vi "REPORT_AUDIT_prepare_results.vi"(11 "REPORT_AUDIT_all_info":T1) -> (3 "Array":string[][](array[string]))   [LabVIEW 2020]
uses:
  typedef/REPORT_AUDIT_all_info.ctl
  GEAR/typedef/REPORT_GEAR_statuses.ctl
  typedef/REPORT_AUDIT_control_index.ctl
  _misc/AULocalize/SubVIs/Get Localized Phrase Compact Interface 1D.vi
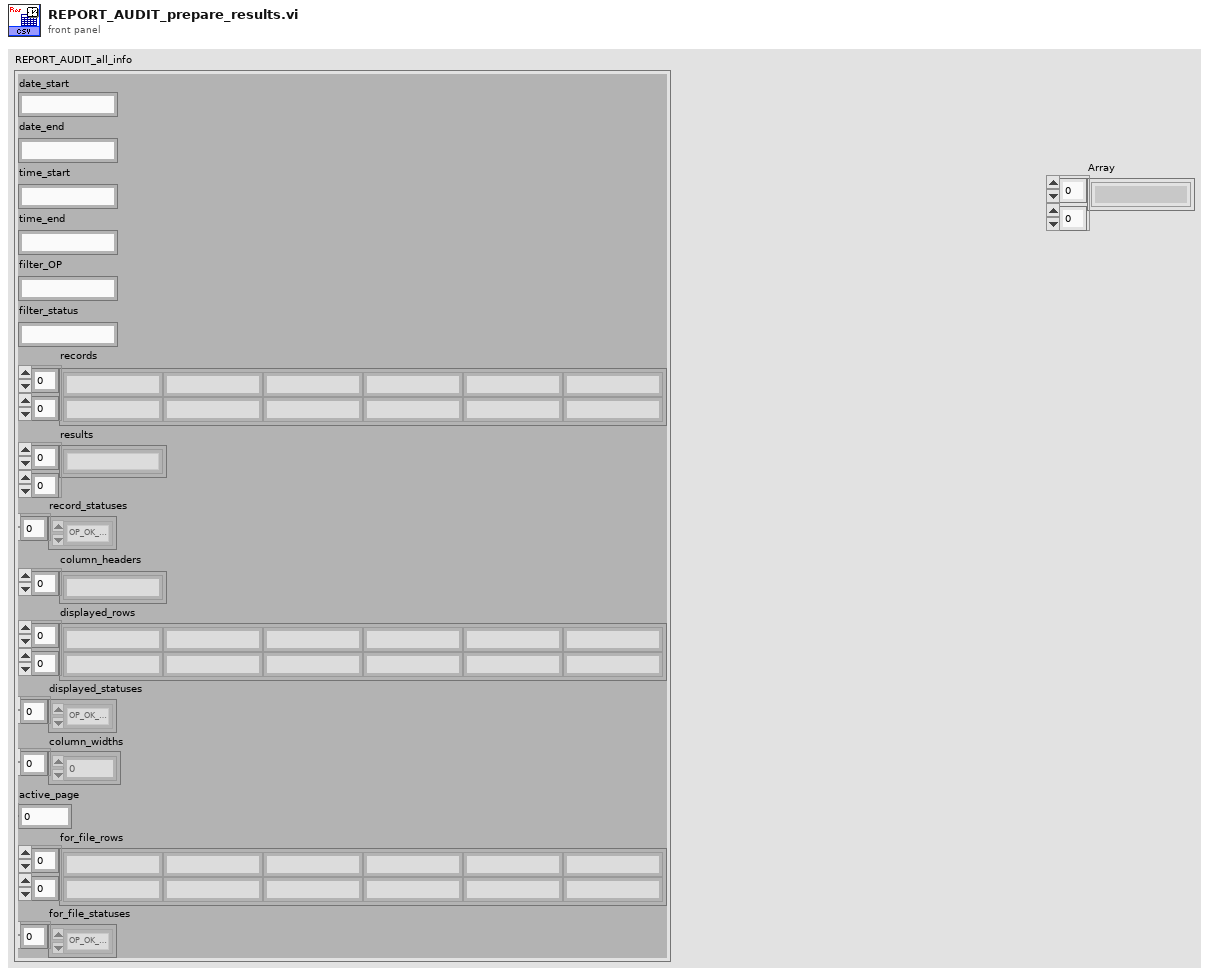
[diagram p1: front panel]
types:
  T1 = typedef "REPORT_AUDIT_all_info.ctl" = cluster{"date_start":string, "date_end":string, "time_start":string, "time_end":string, "filter_OP":string, "filter_status":string, "records":string[][], "results":string[][], "record_statuses":T2[], "column_headers":string[], "displayed_rows":string[][], "displayed_statuses":T2[], "column_widths":i16[], "active_page":i32, "for_file_rows":string[][], "for_file_statuses":T2[]}
  T2 = typedef "REPORT_GEAR_statuses.ctl" = enum16{"OP_OK_hide", "OP_OK_show", "OP_NOK_hide", "OP_NOK_show", "OP_interrupted_hide", "OP_interrupted_show", "OP_in_operation_hide", "OP_in_operation_show", "OP_unexpected_hide", "OP_unexpected_show", "RE_REAL_OK", "RE_REAL_NOK", "RE_STRING", "RE_sub_header", "RE_no_data", "RE_unexpected", "BA_sub_header", "BA_data", "BA_no_data"}
  T3 = typedef "REPORT_AUDIT_control_index.ctl" = enum16{"zeroing", "add_to_index", "get_index"}
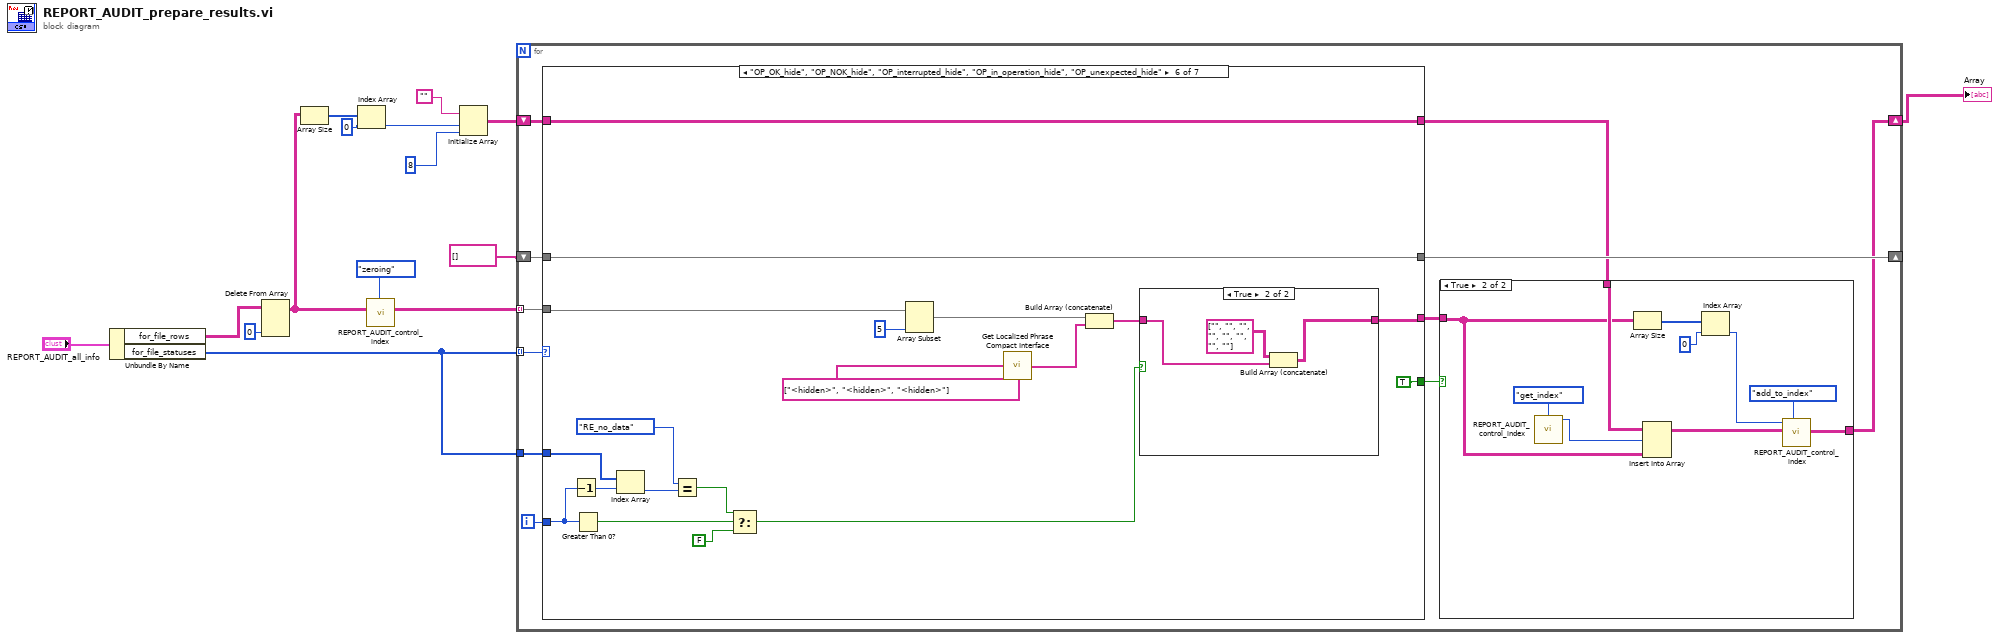
[diagram p0: block diagram]
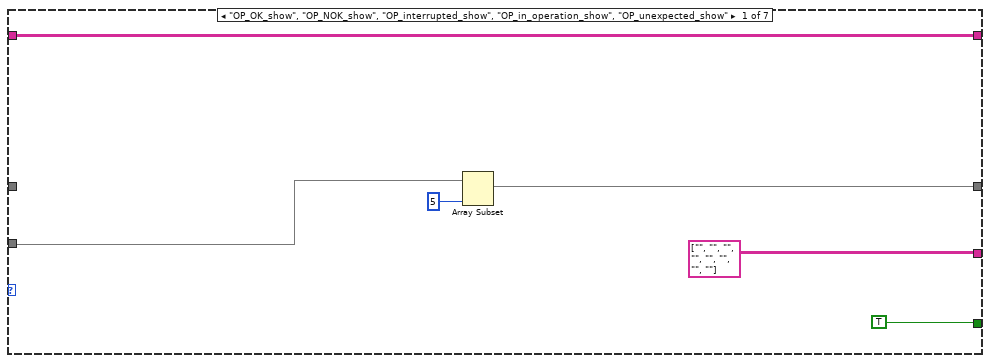
[diagram p3: hidden frame]
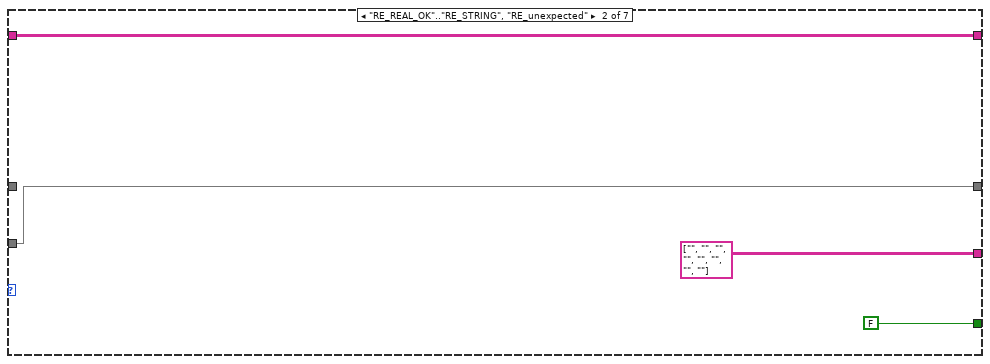
[diagram p4: hidden frame]
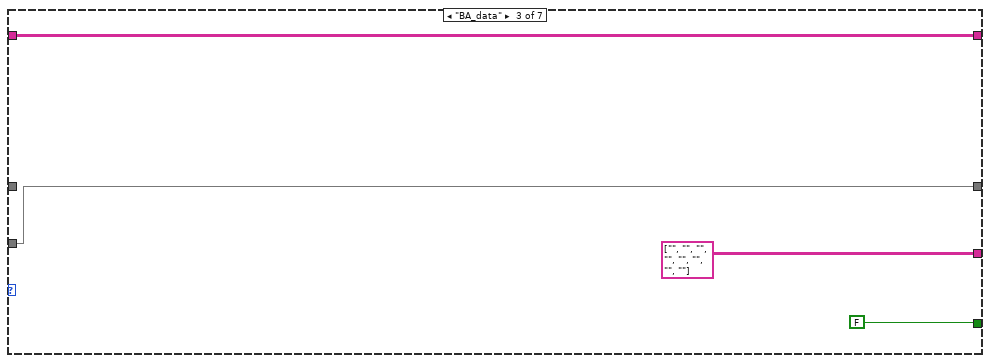
[diagram p5: hidden frame]
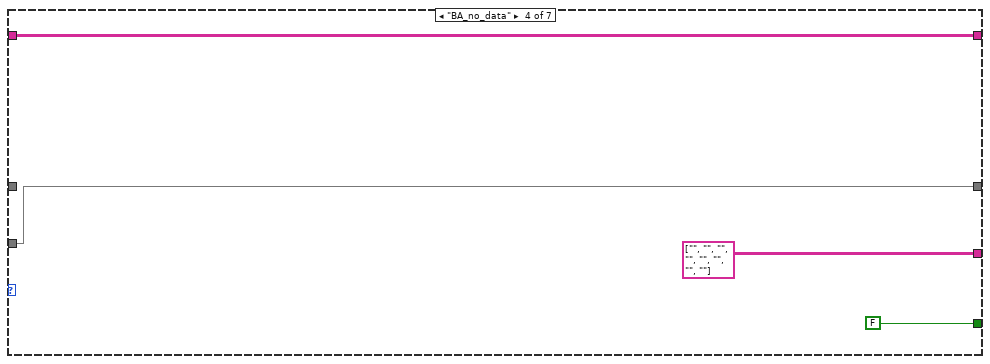
[diagram p6: hidden frame]
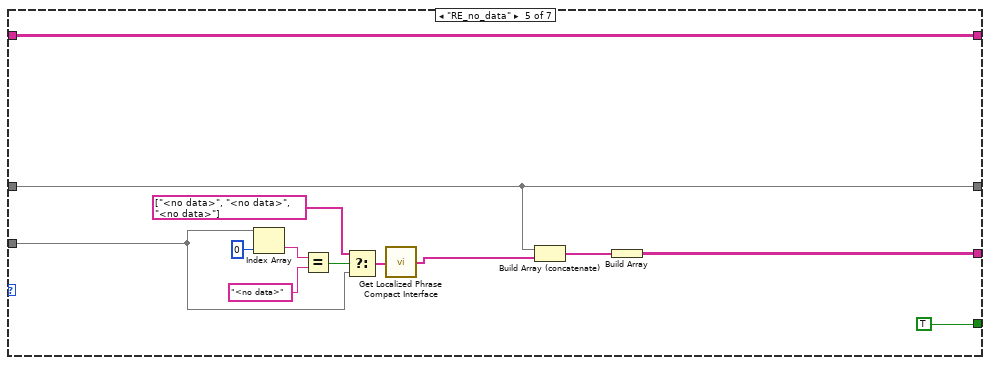
[diagram p7: hidden frame]
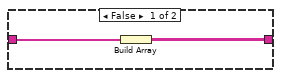
[diagram p8: hidden frame]
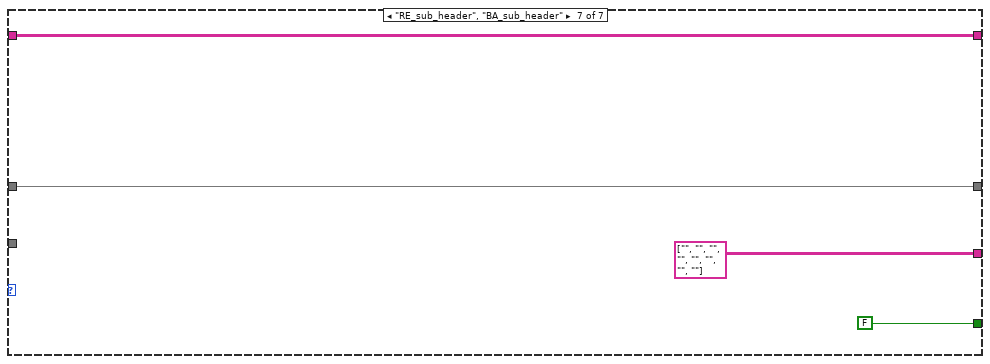
[diagram p9: hidden frame]
diagram:
  n1 = Unbundle By Name("REPORT_AUDIT_all_info") -> ("for_file_rows"=w12:string[][], "for_file_statuses"=w1:T2[])
  n2 = Delete From Array(array=w12, index (col)=0) -> (array with subset deleted=w6:string[][])  [unwired: 2 in, 1 out]
  n3 = Array Size(array=w6) -> (size(s)=w9:i32[])
  n4 = Index Array(array=w9, index=0) -> (element=w10:i32)
  n5 = call "REPORT_AUDIT_control_index.vi"("option"=REPORT_AUDIT_control_index."zeroing" ("Enum"), "array_input"=w6) -> ("array_output"=w5:string[][])  [unwired: 8 in, 1 out]
  n6 = Initialize Array("", w10, 8) -> (w7:string[][])
  n7 = for {
    shift-right: [w26] -> _
    shift-left: string[] [] ("displayed_rows") -> [w23]
    tunnel: w5 -> [w25] mode=indexing
    tunnel: w1 -> [w24] mode=indexing
    shift-right: [w19] -> w3
    shift-left: w7 -> [w21]
    tunnel: w1 -> [w16]
    i -> [w17]
    n8 = case shown="\"OP_OK_hide\", \"OP_NOK_hide\", \"OP_interrupted_hide\", \"OP_in_operation_hide\", \"OP_unexpected_hide\"" w24 {
      tunnel: w25 -> [w43 w44 w48 w52 w61 w86 _]
      tunnel: [w38 w44 w48 w52 w60 w81 w95] -> w26
      tunnel: w23 -> [_ _ _ _ w60 w81 w95]
      tunnel: [string[][] [["", "", "", "", "", "", "", ""]] string[][] [["", "", "", "", "", "", "", ""]] string[][] [["", "", "", "", "", "", "", ""]] string[][] [["", "", "", "", "", "", "", ""]] w58 w69 string[][] [["", "", "", "", "", "", "", ""]]] -> w22
      tunnel: [w40 w47 w51 w53 w59 w82 w96] -> w20
      tunnel: w21 -> [w40 w47 w51 w53 w59 w82 w96]
      tunnel: [TRUE FALSE FALSE FALSE TRUE TRUE FALSE] -> w18
      tunnel: w17 -> [_ _ _ _ _ w77 _]
      tunnel: w16 -> [_ _ _ _ _ w75 _]
      frame "OP_OK_show", "OP_NOK_show", "OP_interrupted_show", "OP_in_operation_show", "OP_unexpected_show" {
        n9 = Array Subset(array=w43, length=5) -> (w38:string[])  [unwired: 1 in]
      }
      frame "RE_REAL_OK".."RE_STRING", "RE_unexpected" {
      }
      frame "BA_data" {
      }
      frame "BA_no_data" {
      }
      frame "RE_no_data" {
        n10 = Index Array(array=w61, index=0) -> (element=w67:string)
        n11 = Equal?(x=w67, y="<no data>" ("String")) -> (x = y?=w65:bool)
        n12 = Select(t=string[] ["<no data>", "<no data>", "<no data>"] ("displayed_rows"), s=w65, f=w61) -> (s? t:f=w63:string[])
        n13 = call-poly "Get Localized Phrase Compact Interface.vi"("Key"=w63) -> ("Translated Phrase"=w62:string[])
        n14 = Build Array (concatenate)(w60, w62) -> (w56:string[])
        n15 = Build Array(w56) -> (w58:string[][])
      }
      frame "OP_OK_hide", "OP_NOK_hide", "OP_interrupted_hide", "OP_in_operation_hide", "OP_unexpected_hide" {
        n16 = Decrement(x=w77) -> (x-1=w76:i32)
        n17 = Greater Than 0?(x=w77) -> (x > 0?=w79:bool)
        n18 = Index Array(array=w75, index=w76) -> (element=w74:T2)
        n19 = Equal?(x=REPORT_GEAR_statuses."RE_no_data" ("REPORT_GEAR_statuses"), y=w74) -> (x = y?=w72:bool)
        n20 = Select(t=w72, s=w79, f=FALSE) -> (s? t:f=w71:bool)
        n21 = Array Subset(array=w86, length=5) -> (w84:string[])  [unwired: 1 in]
        n22 = call-poly "Get Localized Phrase Compact Interface.vi"("Key"=string[] ["<hidden>", "<hidden>", "<hidden>"] ("displayed_rows")) -> ("Translated Phrase"=w83:string[])
        n23 = Build Array (concatenate)(w84, w83) -> (w70:string[])
        n24 = case shown="True" w71 {
          tunnel: w70 -> [w89 w92]
          tunnel: [w88 w90] -> w69
          frame False {
            n25 = Build Array(w89) -> (w88:string[][])
          }
          frame True {
            n26 = Build Array (concatenate)(string[][] [["", "", "", "", "", "", "", ""]], w92) -> (w90:string[][])
          }
        }
      }
      frame "RE_sub_header", "BA_sub_header" {
      }
    }
    n27 = case shown="True" w18 {
      tunnel: w22 -> [_ w31]
      tunnel: [w27 w33] -> w19
      tunnel: w20 -> [w27 w37]
      frame False {
      }
      frame True {
        n28 = call "REPORT_AUDIT_control_index.vi"("option"=REPORT_AUDIT_control_index."get_index" ("Enum")) -> ("index_output"=w35:i32)  [unwired: 9 in, 1 out]
        n29 = Array Size(array=w31) -> (size(s)=w30:i32[])
        n30 = Insert Into Array(array=w37, index (row)=w35, new element=w31) -> (w34:string[][])  [unwired: 1 in]
        n31 = Index Array(array=w30, index=0) -> (element=w28:i32)
        n32 = call "REPORT_AUDIT_control_index.vi"("option"=REPORT_AUDIT_control_index."add_to_index" ("Enum"), "array_input"=w34, "add_value"=w28) -> ("array_output"=w33:string[][])  [unwired: 7 in, 1 out]
      }
    }
  }
  "Array" <- w3
